vi "Dashboard Main.vi"() -> ()   [LabVIEW 2014]
uses:
  <vilib>/event_ctls.llb/eventvkey.ctl
  <vilib>/Rock Robotics/WPI/Dashboard/WPI_DashboardLogging Global.vi
  <vilib>/Utility/config.llb/Write Key (String).vi
  <vilib>/Utility/config.llb/Write Key (I32).vi
  <vilib>/Utility/config.llb/NI_LVConfig.lvlib
panel:
  in  "TCP":refnum<k5>
  in  "Rec Mode":enum32{"Stop", "Record", "Playback"}(radio)
  in  "Vision":u16(ring) items=["Camera Off", "USB Camera SW", "USB Camera HW", "IP Camera"]
  out "Camera IP":string
  out "Image Message":string="Timeout in Camera Communications"
  in  "Dashboard Tab":T1(tab)
  in  "Camera Settings":T2={"Frame Rate"=30, "Compression"=30, "Size"=1} {"Frame Rate" scale=1.0..30.0; "Size" items=["640x480", "320x240", "160x120"]}
  out "MotorChart R":cluster{"Numeric":dbl, "Numeric":dbl}(graph)
  out "MotorChart L":T3(graph)
  out "MotorSliders R":cluster{"MotorSlide1":dbl, "MotorSlide2":dbl} {"MotorSlide2" scale=-1.0..1.0 scale format="%#_2e"; "MotorSlide1" scale=-1.0..1.0 scale format="%#_2e"}
  out "MotorSliders L":T4 {"MotorSlide4 2" scale=0.0..14.0 scale format="%#_2e"; "MotorSlide2" scale=-1.0..1.0 scale format="%#_2e"; "MotorSlide1" scale=-1.0..1.0 scale format="%#_2e"}
  out "Gyro":dbl(knob) scale=0.0..360.0
  out "JS1 Z":dbl(slide) scale=-1.0..1.0 scale format="%#_2e"
  out "JS1 Graph":cluster{"X":dbl, "Y":dbl}[](graph)
  out "JS1 Buttons":T5
  out "JS2 Z":dbl(slide) scale=-1.0..1.0 scale format="%#_2e"
  out "JS2 Graph":cluster{"X":dbl, "Y":dbl}[](graph)
  out "JS2 Buttons":T5
  out "Mode":T6(ring)=enum."Auto Disabled"
  in  "DB Camera Config":bool
  out "fps":dbl format="%#.1g"
  out "Mbps":dbl format="%#.1g"
  out "Mbps 2":bool
  in  "DB/String 9":string
  in  "DB/String 8":string
  in  "DB/String 7":string
  in  "DB/String 6":string
  in  "DB/String 5":string
  in  "DB/String 4":string
  in  "DB/String 3":string
  in  "DB/String 2":string
  in  "DB/String 1":string
  in  "DB/String 0":string
  in  "DB/Slider 0":dbl(slide) scale=0.0..5.0
  in  "DB/Slider 1":dbl(slide) scale=0.0..5.0
  in  "DB/Slider 2":dbl(slide) scale=0.0..5.0
  in  "DB/Slider 3":dbl(slide) scale=0.0..5.0
  out "DB/LED 3":bool
  out "DB/LED 2":bool
  out "DB/LED 1":bool
  out "DB/LED 0":bool
  in  "DB/Button 3":bool
  in  "DB/Button 2":bool
  in  "DB/Button 1":bool
  in  "DB/Button 0":bool caption="New Name"
  in  "Boolean 2":bool
  in  "Upload code":bool
  out "Speed Value":dbl
  in  "Speed":string
  out "Deadzone Value":dbl
  in  "Deadzone":string
  in  "Upload Code":bool
  in  "Test Slider":dbl(slide) scale=0.0..100.0 scale format="%#_3g"
  in  "On/Off":bool caption="Solenoid"
  in  "Test Name":u16(ring) items=["Select the test to run...", "Example Test", "-------------------------------", "List of tests is built in robot code.", "Replace with your own automated tests."]
  in  "Test Tree":string(tree)
  in  "Motor":cluster{"Value":dbl, "Enable":bool} {"Value" scale=-1.0..1.0 scale format="%#_3g"}
  out "Progress":T7 {"Test Progress" scale=0.0..100.0}
  in  "Rev/Fwd":cluster{"Forward":bool, "Reverse":bool}
  in  "Test Ring":u16(ring) items=["Monochrome", "Color"]
  in  "Listbox":i32(listbox)
  out "Tree":string(tree)
  out "Camera Image":T8(plugin-control)
  out "Boolean":bool
  # "Left"
  # "Front"
  # "Right"
  # "Battery"
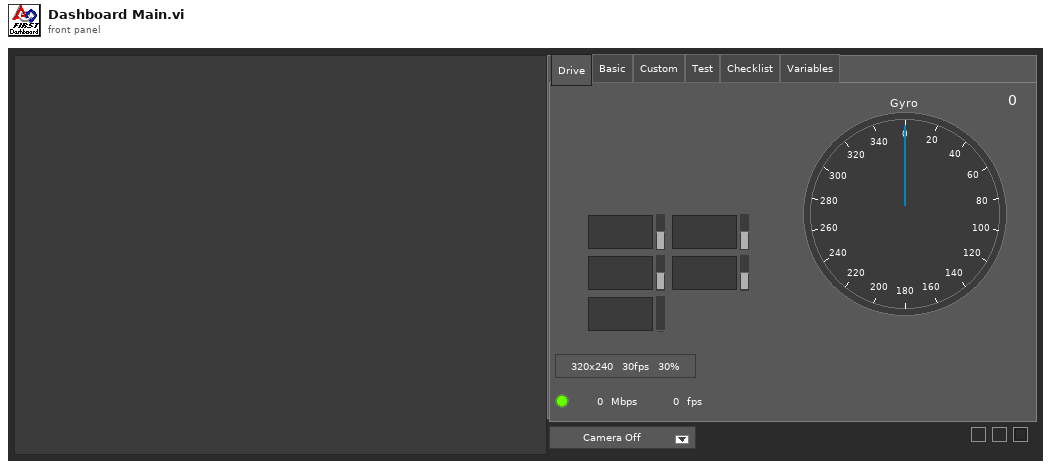
[diagram p1: front panel]
types:
  T1 = enum32{"Drive", "Basic", "Custom", "Test", "Checklist", "Variables"}
  T2 = cluster{"Frame Rate":i32, "Compression":i32, "Size":u16}
  T3 = cluster{"Numeric":dbl, "Numeric":dbl, "Battery V":dbl}
  T4 = cluster{"MotorSlide1":dbl, "MotorSlide2":dbl, "MotorSlide4 2":dbl}
  T5 = cluster{bool, bool, bool, bool, bool, bool, bool, bool, bool, bool, bool, bool}
  T6 = enum8{"Tele-Op Disabled", "Tele-Op Enabled", "Auto Disabled", "Auto Enabled", "Test Disabled", "Test Enabled", "Disconnected", "No Code", "E-Stop"}
  T7 = cluster{"Test Progress":u8, "Test Progress Text":string}
  T8 = typedef "IMAQ Image.ctl" = refnum<image>
  T9 = typedef "Image Type" = u32
  T10 = cluster{"Camera Image":refnum<vi>, "Dashboard Tab":refnum<vi>, "Boolean":refnum<vi>, "Vision":refnum<vi>, "Rec Mode":refnum<vi>, "Test Slider":refnum<vi>, "On/Off ":refnum<vi>, "Test Ring":refnum<vi>, "Rev/Fwd":refnum<vi>, "Test Name":refnum<vi>, "Motor":refnum<vi>, "Progress":refnum<vi>, "CheckList":refnum<vi>, "Tree":refnum<vi>, "Test Tree":refnum<vi>}
  T11 = cluster{"Error Strings":string, "Disable Counts":cluster{u16, u16}, "Rail Faults":cluster{u16, u16, u16}, "Robot IP":string, "DB Mode":u8, "Event Info":cluster{"Name":string, "Type":u8, "Number":u16, "Replay":u8}, "Camera Addr":string}
  T12 = cluster{"Storage":cluster{"Disk Free":u64, "RAM Block":u32, "RAM free":u32}, "CPU Utilization":cluster{"CPU % ISR":sgl, "CPU % Time Crit":sgl, "CPU % Timed Str":sgl, "CPU % High":sgl, "CPU % Above":sgl, "CPU % Normal":sgl, "CPU % Low":sgl}, "CAN":cluster{"% Bus Utilization":sgl, "Bus Off Cnt":u32, "TX_FIFO Full Cnt":u32, "Receive Error Cnt":u8, "Transmit Error Cnt":u8}, "HID":cluster{"HID Outputs":u32, "Rumble Low":u16, "Rumble High":u16}[]}
  T13 = cluster{"Status bits":cluster{"Test Mode":bool, "Autonomous":bool, "Enabled":bool, "Code Start":bool, "Brownout":bool, "Reserved 2":bool, "Reserved 3":bool, "E-Stop":bool}, "Code Trace":cluster{"Disabled":bool, "TeleOp":bool, "Auto":bool, "Test":bool}, "Controller Type":enum16{"unknown", "cRIO", "roboRio"}, "Code?":enum16{"unknown", "noCode", "code"}, "Battery V":dbl}
  T14 = cluster{"Control Bits":cluster{"TestMode":bool, "Autonomous":bool, "Enabled":bool, "FMS Present":bool, bool, bool, bool, "E-Stop":bool}, "Team Station ":u8, "Countdown":sgl, "Joystick Values":cluster{"Axes":dbl[], "Buttons":bool[], "POVs":i16[]}[]}
  T15 = cluster{"Axes":dbl[], "Buttons":bool[], "POVs":i16[]}[]
  T16 = cluster{"Axes":dbl[], "Buttons":bool[], "POVs":i16[]}
  T17 = cluster{"Buttons[0]":bool, "Buttons[1]":bool, "Buttons[2]":bool, "Buttons[3]":bool, "Buttons[4]":bool, "Buttons[5]":bool, "Buttons[6]":bool, "Buttons[7]":bool, "Buttons[8]":bool, "Buttons[9]":bool, "Buttons[10]":bool, "Buttons[11]":bool}
  T18 = typedef "NI_LVConfig.lvlib/Config Data RefNum.ctl" = refnum<k1>
  T19 = cluster{"Operation":enum16{"Update", "Clear"}, "Color Box":u32}[]
  T20 = typedef "eventvkey.ctl" = enum16{"ASCII", "Enter", "Return", "Shift", "Ctrl", "Alt", "Cmd", "Opt", "Caps", "NumLock", "Clear", "Break", "Up", "Down", "Left", "Right", "Insert", "Delete", "Home", "End", "PageUp", "PageDown", "Escape", "Help", "Pause", "ScrollLock", "F1", "F2", "F3", "F4", "F5", "F6", "F7", "F8", "F9", "F10", "F11", "F12", "F13", "F14", "F15", "F16", "F17", "F18", "F19", "F20", "F21", "F22", "F23", "F24", "Play", "VolumeUp", "VolumeDown", "Mute", "Two Byte Char"}
  T21 = cluster{"Image Size":bool, "Image Type":bool, "Pixel Value":bool, "ROI Information":bool, "Zoom Factor":bool}
  T22 = enum8{"Enabled", "Disabled", "Disabled and Grayed Out"}
  T23 = cluster{"Operation":enum16{"Update", "Clear"}, "Color Box":u32}
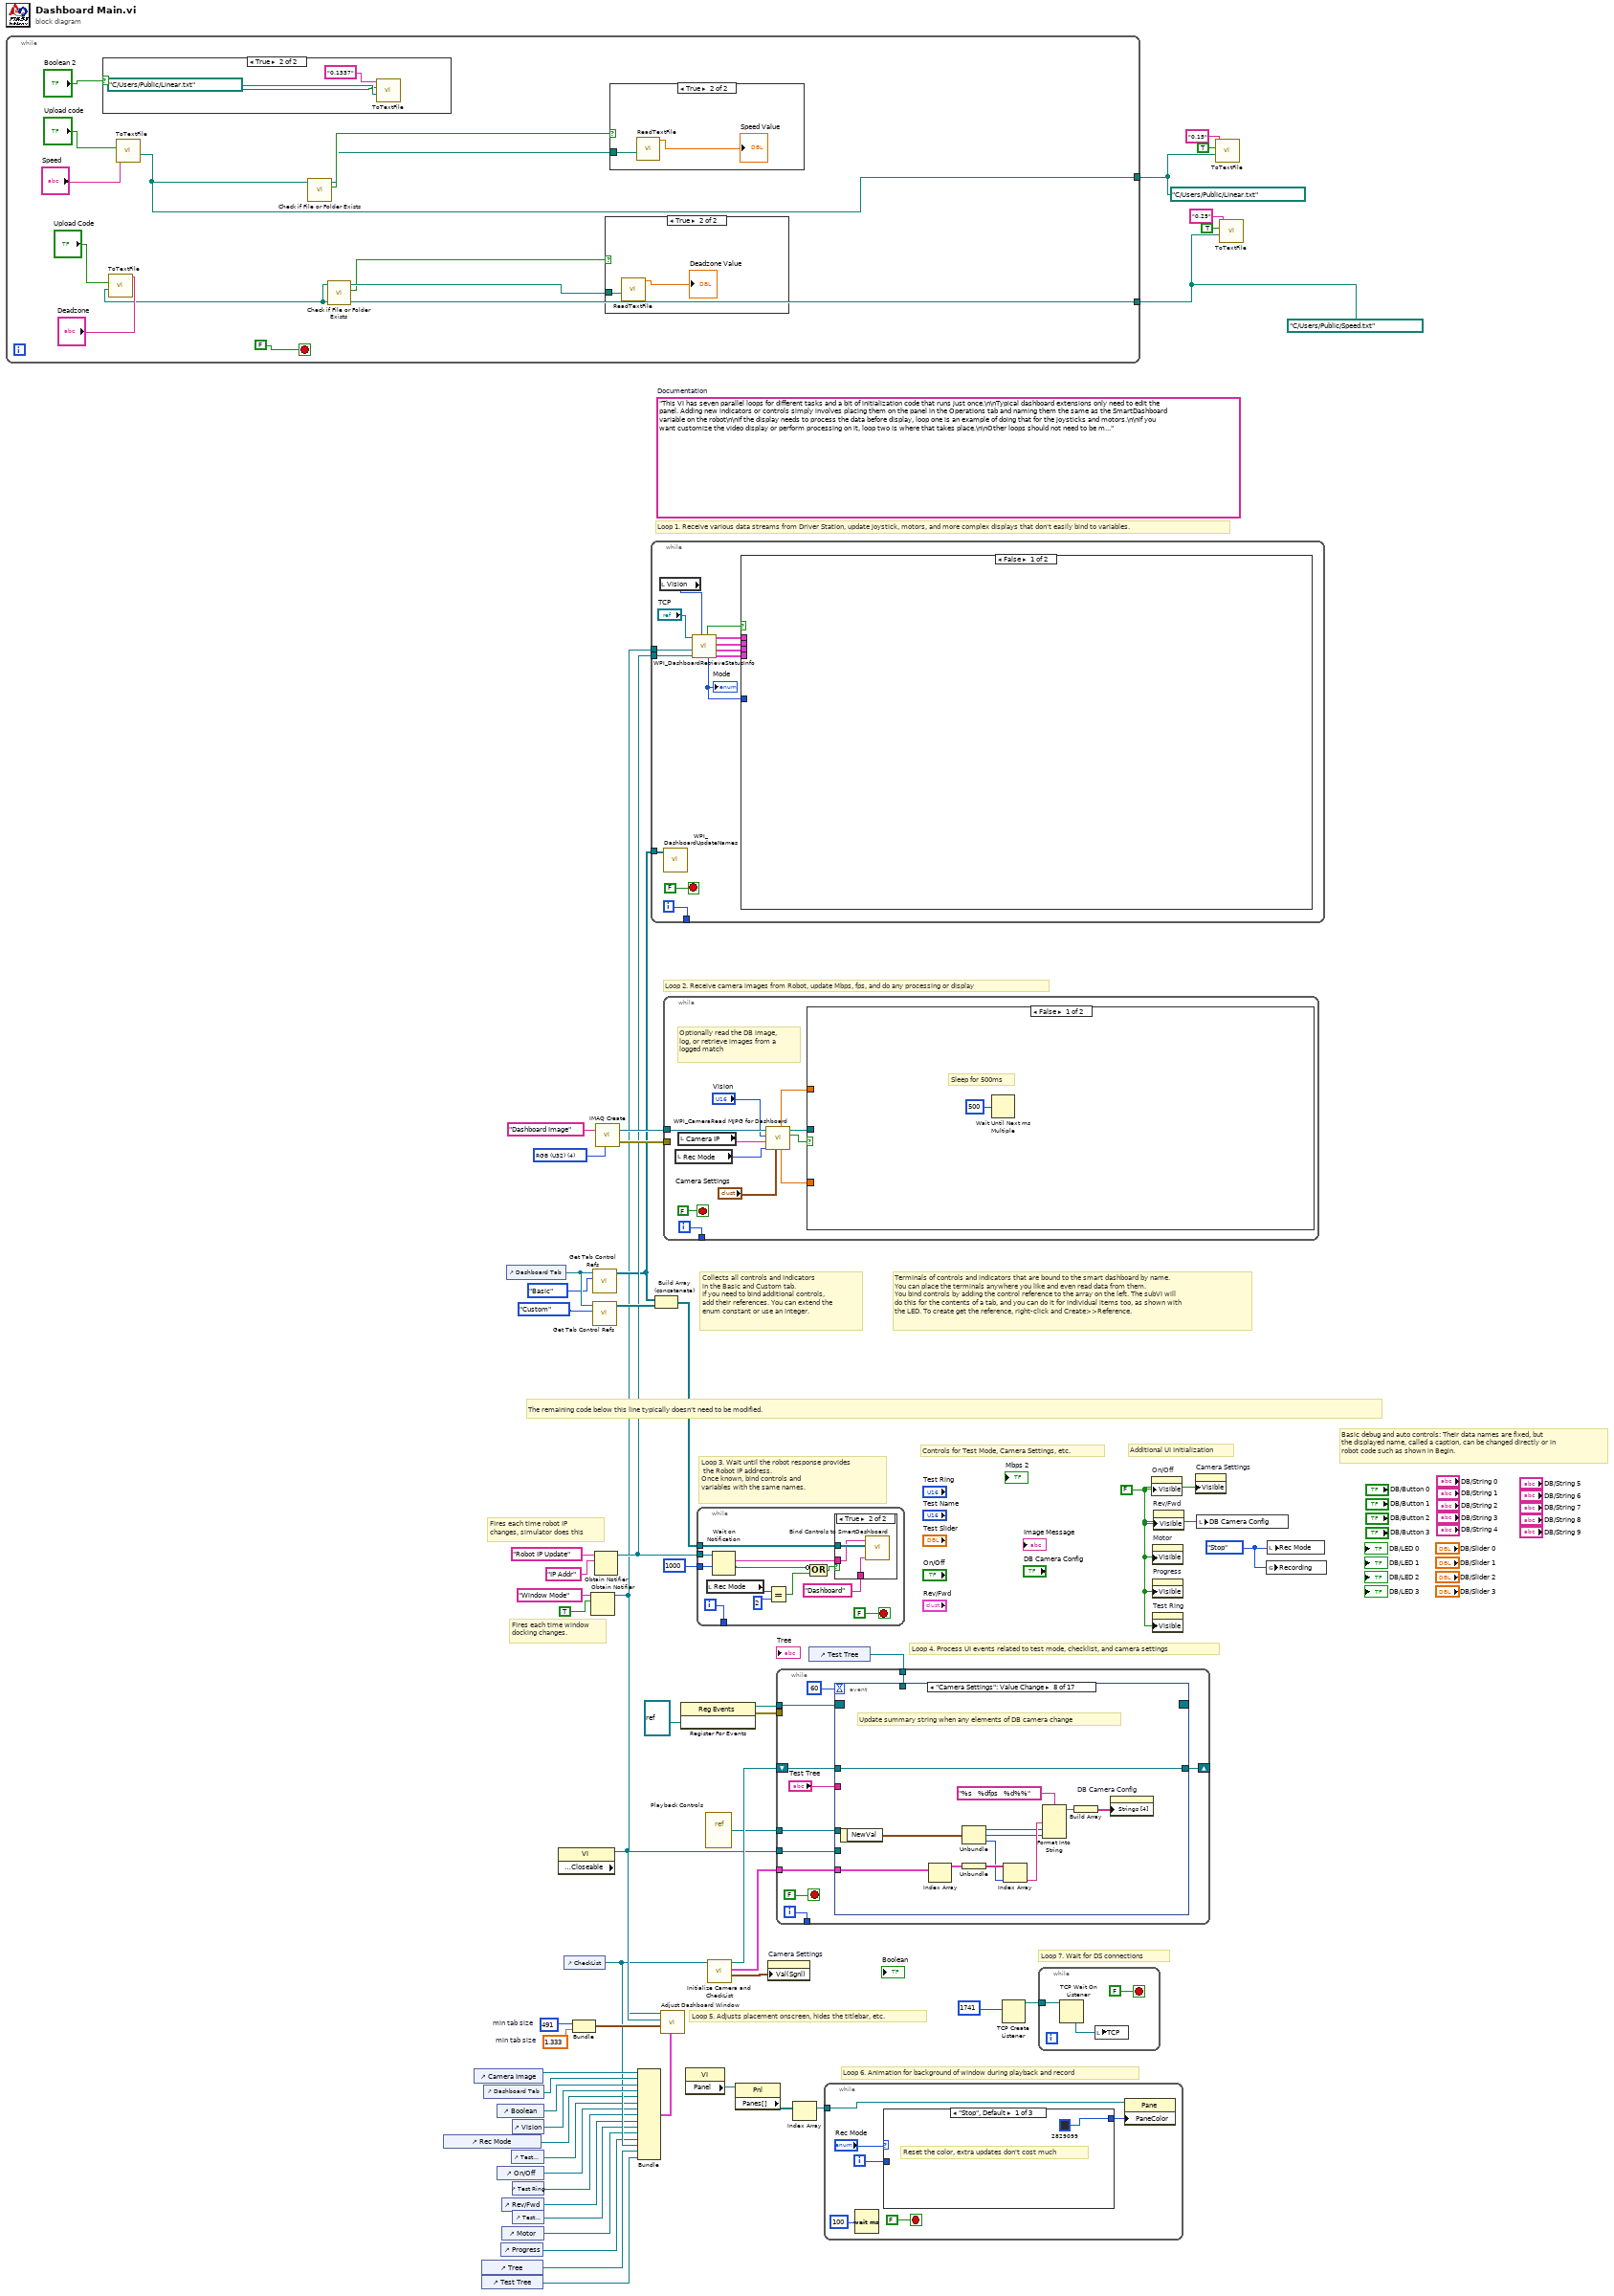
[diagram p0: block diagram]
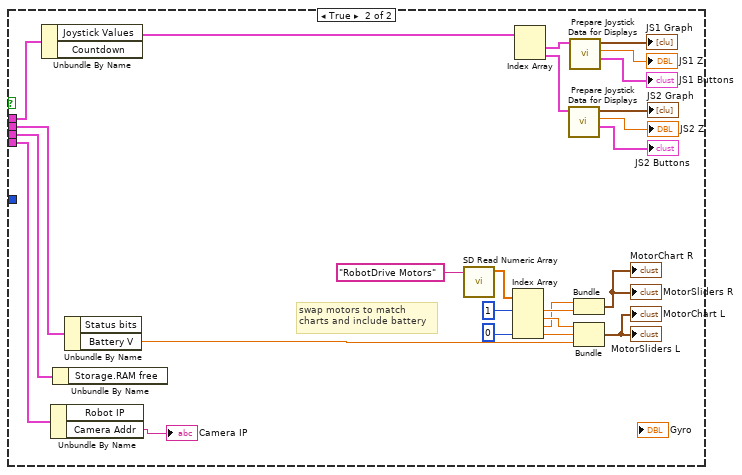
[diagram p5: hidden frame]
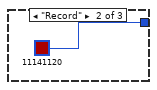
[diagram p6: hidden frame]
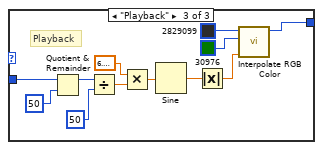
[diagram p7: hidden frame]
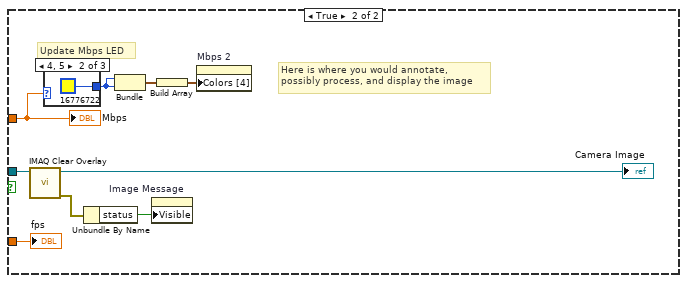
[diagram p9: hidden frame]
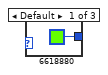
[diagram p10: hidden frame]
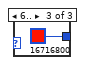
[diagram p11: hidden frame]
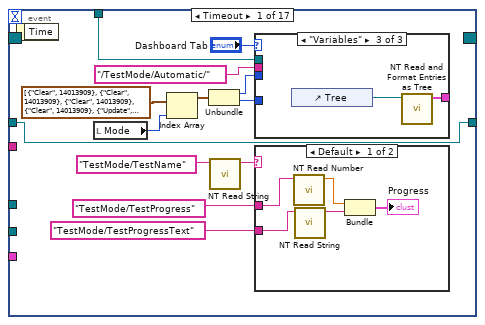
[diagram p12: hidden frame]
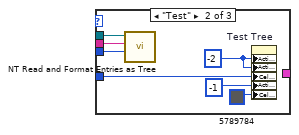
[diagram p14: hidden frame]
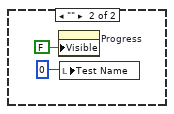
[diagram p15: hidden frame]
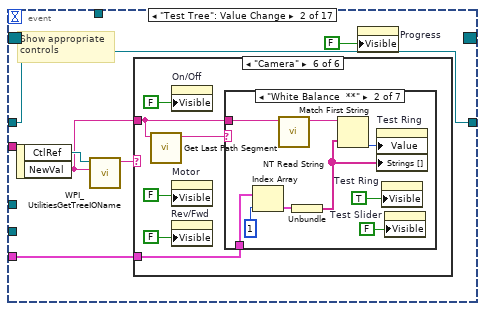
[diagram p16: hidden frame]
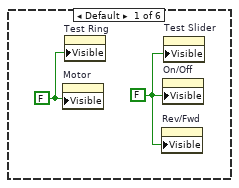
[diagram p17: hidden frame]
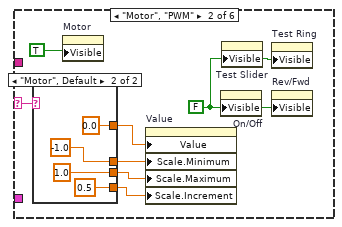
[diagram p18: hidden frame]
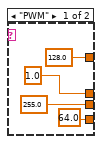
[diagram p19: hidden frame]
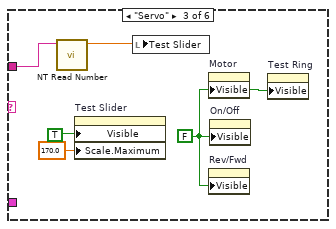
[diagram p20: hidden frame]
diagram:
  w2 = path "C:/Users/Public/Linear.txt" ("file path (use dialog)")
  w1 = path "C:/Users/Public/Speed.txt" ("file path (use dialog)")
  w30 = 491  # min tab size
  w29 = 1.333  # min tab size
  w38 = enum32{"Stop", "Record", "Playback"}."Stop" ("Rec Mode")
  w12 = FALSE ("Visible")
  (unwired) "This VI has seven parallel loops for different tasks and a bit of initialization code that runs just once.\n\nTypical dashboard extensions only need to edit the panel. Adding new indicators or controls simply involves placing them on the panel in the Operations tab and naming them the same as the SmartDashboard variable on the robot\n\nIf the display needs to process the data before display, loop one is an example of doing that for the joysticks and motors.\n\nIf you want customize the video display or perform processing on it, loop two is where that takes place.\n\nOther loops should not need to be modified. They are pretty standard, and document the task they perform."  # Documentation
  w58 = T9 4 items=["Grayscale (U8)", "Grayscale (I16)", "Grayscale (SGL)", "Complex (CSG)", "RGB (U32)", "HSL (U32)", "RGB (U64)"] ("Image Type")
  # "Loop 7. Wait for DS connections"
  # "Basic debug and auto controls: Their data names are fixed, but\nthe displayed name, called a caption, can be changed directly or in\nrobot code such as shown in Begin."
  # "Controls for Test Mode, Camera Settings, etc."
  # "Additional UI Initialization"
  # "Loop 6. Animation for background of window during playback and record"
  # "Fires each time robot IP\nchanges, simulator does this"
  # "Fires each time window\ndocking changes."
  # "Collects all controls and indicators\nin the Basic and Custom tab.\nIf you need to bind additional controls,\nadd their references. You can extend the\nenum constant or use an integer."
  # "The remaining code below this line typically doesn't need to be modified."
  # "Loop 4. Process UI events related to test mode, checklist, and camera settings"
  # "Terminals of controls and indicators that are bound to the smart dashboard by name.\nYou can place the terminals anywhere you like and even read data from them.\nYou bind controls by adding the control reference to the array on the left. The subVI will\ndo this for the contents of a tab, and you can do it for individual items too, as shown with\nthe LED. To create get the reference, right-click and Create>>Reference."
  # "Loop 3. Wait until the robot response provides\n the Robot IP address.\nOnce known, bind controls and\nvariables with the same names."
  # "Loop 5. Adjusts placement onscreen, hides the titlebar, etc."
  # "Loop 1. Receive various data streams from Driver Station, update joystick, motors, and more complex displays that don't easily bind to variables."
  # "Loop 2. Receive camera images from Robot, update Mbps, fps, and do any processing or display"
  n1 = while {
    tunnel: w2 -> [w60]
    tunnel: w1 -> [w59]
    stop <- FALSE stop-if-true
    n2 = case shown="True" "Boolean 2" {
      selector: "Boolean 2" -> [_ w76]
      frame False {
      }
      frame True {
        n3 = call "ToTextFile.vi"("file path (use dialog)"=path "C:/Users/Public/Linear.txt", "Boolean"=w76, "String"="0.1337") -> ()  [unwired: 8 in, 1 out]
      }
    }
    n4 = call "ToTextFile.vi"("file path (use dialog)"=w59, "Boolean"="Upload Code", "String"="Deadzone") -> ()  [unwired: 8 in, 1 out]
    n5 = call "ToTextFile.vi"("file path (use dialog)"=w60, "Boolean"="Upload code", "String"="Speed") -> ()  [unwired: 8 in, 1 out]
    n6 = call <vilib>:"Check if File or Folder Exists.vi"("path"=w60) -> ("file or folder exists?"=w64:bool, "dup path"=w63:path)  [unwired: 8 in, 1 out]
    n7 = call <vilib>:"Check if File or Folder Exists.vi"("path"=w59) -> ("file or folder exists?"=w61:bool, "dup path"=w62:path)  [unwired: 8 in, 1 out]
    n8 = case shown="True" w61 {
      tunnel: w62 -> [_ w71]
      frame False {
      }
      frame True {
        n9 = call "ReadTextFile.vi"("file (use dialog)"=w71) -> ("Double"=→"Deadzone Value":dbl)  [unwired: 9 in, 1 out]
      }
    }
    n10 = case shown="True" w64 {
      tunnel: w63 -> [_ w73]
      frame False {
      }
      frame True {
        n11 = call "ReadTextFile.vi"("file (use dialog)"=w73) -> ("Double"=→"Speed Value":dbl)  [unwired: 9 in, 1 out]
      }
    }
  }
  n12 = control-ref of="Rec Mode"() -> (w18:refnum<vi>)
  n13 = control-ref of="Camera Image"() -> (w33:refnum<vi>)
  n14 = control-ref of="Tree"() -> (w22:refnum<vi>)
  n15 = control-ref of="Test Tree"() -> (w21:refnum<vi>)
  n16 = control-ref of="Dashboard Tab"() -> (w32:refnum<vi>)
  n17 = control-ref of="Boolean"() -> (w27:refnum<vi>)
  n18 = control-ref of="On/Off"() -> (w16:refnum<vi>)
  n19 = control-ref of="Progress"() -> (w13:refnum<vi>)
  n20 = control-ref of="Rev/Fwd"() -> (w14:refnum<vi>)
  n21 = control-ref of="Motor"() -> (w19:refnum<vi>)
  n22 = control-ref of="Dashboard Tab"() -> (w36:refnum<vi>)
  n23 = control-ref of="Test Slider"() -> (w17:refnum<vi>)
  n24 = control-ref of="Vision"() -> (w31:refnum<vi>)
  n25 = control-ref of="Test Ring"() -> (w15:refnum<vi>)
  n26 = control-ref of="Test Name"() -> (w20:refnum<vi>)
  n27 = property class="VI" props=["Front Panel.Closeable"]() -> (reference out=w37:refnum<vi>)  [unwired: 2 in, 2 out]
  n28 = control-ref of="CheckList"() -> (w23:refnum<vi>)
  n29 = Bundle("min tab size"=w30, "min tab size"=w29) -> (w28:cluster{"min tab size":i32, "min tab size":dbl})  [unwired: 1 in]
  n30 = Obtain Notifier(name (unnamed)="Window Mode", notification data type=TRUE) -> (notifier out=w9:refnum<notifier>)  [unwired: 2 in, 2 out]
  n31 = call <vilib>:"Get Tab Control Refs.vi"("Page Index"=T1."Basic" ("Dashboard Tab"), "TabControl in"=w36) -> ("ControlsOnPage"=w10:refnum<vi>[])  [unwired: 9 in]
  n32 = call <vilib>:"Get Tab Control Refs.vi"("Page Index"=T1."Custom" ("Dashboard Tab"), "TabControl in"=w36) -> ("ControlsOnPage"=w35:refnum<vi>[])  [unwired: 9 in]
  n33 = Obtain Notifier(name (unnamed)="Robot IP Update", notification data type="IP Addr" ("name (unnamed)")) -> (notifier out=w11:refnum<notifier>)  [unwired: 2 in, 2 out]
  n34 = call "IMAQ Create"("Image Name"="Dashboard Image", "Image Type"=w58) -> ("New Image"=w56:T8, "error out"=w55:errorcluster)  [unwired: 2 in, 1 out]
  n35 = Bundle("Camera Image"=w33, "Dashboard Tab"=w32, "Boolean"=w27, "Vision"=w31, "Rec Mode"=w18, "Test Slider"=w17, "On/Off"=w16, "Test Ring"=w15, "Rev/Fwd"=w14, "Test Name"=w20, "Motor"=w19, "Progress"=w13, "CheckList"=w23, "Tree"=w22, "Test Tree"=w21) -> (w24:T10)  [unwired: 1 in]
  n36 = while {
    tunnel: [w89] -> _
    tunnel: w11 -> [w83]
    tunnel: w10 -> [w82]
    tunnel: w9 -> [w78]
    i -> [w89]
    stop <- FALSE stop-if-true
    n37 = local read "Vision"() -> (w80:u16)
    n38 = call <vilib>:"WPI_DashboardUpdateNames.vi"("Controls on Tab"=w82) -> ()  [unwired: 11 in]
    n39 = call <vilib>:"WPI_DashboardRetrieveStatusInfo.vi"("Vision"=w80, "Binding Refnum"=w83, "Window Mode Notifier"=w78, "TCP Cnx"="TCP") -> ("Power and Errors"=w84:T11, "Robot Metrics"=w87:T12, "Status Info"=w88:T13, "Control Info"=w85:T14, "Robot Mode"=w81:T6, "Process?"=w86:bool)  [unwired: 2 in]
    "Mode" <- w81
    n40 = case shown="False" w86 {
      tunnel: w88 -> [_ w115]
      tunnel: w87 -> [_ w114]
      tunnel: w85 -> [_ w113]
      tunnel: w84 -> [_ w112]
      tunnel: w81 -> [_ _]
      frame False {
      }
      frame True {
        # "swap motors to match\ncharts and include battery"
        n41 = Unbundle By Name(w113) -> ("Joystick Values"=w100:T15)  [unwired: 1 out]
        n42 = Unbundle By Name(w112) -> ("Camera Addr"=→"Camera IP":string)  [unwired: 1 out]
        n43 = Unbundle By Name(w114) -> ()  [unwired: 1 out]
        n44 = Unbundle By Name(w115) -> ("Battery V"=w101:dbl)  [unwired: 1 out]
        n45 = call <vilib>:"SD Read Numeric Array.vi"("Name"="RobotDrive Motors") -> ("Numeric Array"=w103:dbl[])  [unwired: 8 in, 2 out]
        n46 = Index Array(array=w103, index #1=1, index #4=0) -> (element #1=w107:dbl, element #2=w108:dbl, element #3=w106:dbl, element #4=w111:dbl)  [unwired: 2 in]
        n47 = Index Array(array=w100) -> (element #1=w99:T16, element #2=w94:T16)  [unwired: 2 in]
        n48 = call "Prepare Joystick Data for Displays.vi"("Joystick Values"=w94) -> ("Buttons"=→"JS2 Buttons":T17, "Z Axis"=→"JS2 Z":dbl, "Cartesian Data"=→"JS2 Graph":cluster{"X axis":dbl, "X axis":dbl}[])  [unwired: 8 in]
        n49 = call "Prepare Joystick Data for Displays.vi"("Joystick Values"=w99) -> ("Buttons"=→"JS1 Buttons":T17, "Z Axis"=→"JS1 Z":dbl, "Cartesian Data"=→"JS1 Graph":cluster{"X axis":dbl, "X axis":dbl}[])  [unwired: 8 in]
        n50 = Bundle("Numeric"=w106, "Numeric"=w107) -> (→"MotorChart R" →"MotorSliders R":cluster{"Numeric":dbl, "Numeric":dbl})  [unwired: 1 in]
        n51 = Bundle("Numeric"=w108, "Numeric"=w111, "Battery V"=w101) -> (→"MotorChart L" →"MotorSliders L":T3)  [unwired: 1 in]
      }
    }
  }
  n52 = Build Array (concatenate)(w10, w35) -> (w34:refnum<vi>[])
  n53 = call "Adjust Dashboard Window.vi"("Sizing Refnums"=w24, "Size Constraints"=w28, "VI"=w37, "Notifier in"=w9) -> ()  [unwired: 8 in]
  n54 = while {
    tunnel: w56 -> [w124]
    tunnel: w55 -> [_]
    tunnel: [w125] -> _
    i -> [w125]
    stop <- FALSE stop-if-true
    # "Optionally read the DB image,\nlog, or retrieve images from a\nlogged match"
    n55 = local read "Rec Mode"() -> (w118:enum32{"Stop", "Record", "Playback"})
    n56 = local read "Camera IP"() -> (w116:string)
    n57 = call <vilib>:"WPI_CameraRead MJPG for Dashboard.vi"("Camera Settings"="Camera Settings", "Rec Mode"=w118, "Camera IP"=w116, "Camera Mode"="Vision", "Refnum in"=w124) -> ("Active"=w122:bool, "Refnum out"=w123:T8, "FPS"=w121:dbl, "Bandwidth (Mbps)"=w120:dbl)  [unwired: 3 in]
    n58 = case shown="False" w122 {
      tunnel: w123 -> [_ w131]
      tunnel: w120 -> [_ w130]
      tunnel: w121 -> [_ w128]
      frame False {
        # "Sleep for 500ms"
        n59 = Wait Until Next ms Multiple(millisecond multiple=u32 500) -> ()  [unwired: 1 out]
      }
      frame True {
        # "Here is where you would annotate,\npossibly process, and display the image"
        # "Update Mbps LED"
        n60 = call "IMAQ Clear Overlay"("Image"=w131) -> ("error out"=w135:errorcluster, "Image Out"=→"Camera Image":T8)  [unwired: 2 in, 7 out]
        n61 = case shown="4, 5" w130 {
          tunnel: [u32 6618880 ("Color Box") u32 16776722 ("Color Box") u32 16716800 ("Color Box")] -> w132
          frame Default {
          }
          frame 4, 5 {
          }
          frame 6.. {
          }
        }
        n62 = Unbundle By Name(w135) -> ("status"=w136:bool)
        n63 = Bundle("Color Box"=w132, "Color Box"=w132) -> (w134:cluster{"Color Box":u32, "Color Box":u32})  [unwired: 1 out]
        n64 = property on="Image Message" class="Str"("Visible"=w136) -> ()  [unwired: 2 in, 2 out]
        n65 = Build Array(w134) -> (w133:cluster{"Color Box":u32, "Color Box":u32}[])
        n66 = property on="Mbps 2" class="Bool (strict)"("Colors [4]"=w133) -> ()  [unwired: 2 in, 2 out]
        "Mbps" <- w130
        "fps" <- w128
      }
    }
  }
  n67 = register-events(refnum<vi> refnum) -> (reference out=w42:refnum<event-registration>, error out=w41:errorcluster)  [unwired: 2 in]
  n68 = property class="VI"() -> ("Panel"=w45:refnum<vi>)  [unwired: 2 in, 2 out]
  n69 = while {
    tunnel: w34 -> [w151]
    tunnel: w11 -> [w149]
    tunnel: [w147] -> _
    tunnel: u32 1000 ("milliseconds to wait") -> [w146]
    i -> [w147]
    stop <- FALSE stop-if-true
    n70 = local read "Rec Mode"() -> (w142:enum32{"Stop", "Record", "Playback"})
    n71 = Wait on Notification(notifier=w149, timeout in ms (-1)=w146) -> (notification=w148:string, timed out?=w144:bool)  [unwired: 2 in, 2 out]
    n72 = Equal?(x=w142, y=u16 2 ("Rec Mode")) -> (x = y?=w143:bool)
    n73 = Compound Arithmetic op=OR(invert w144, w143) -> (w145:bool)
    n74 = case shown="True" w145 {
      tunnel: w151 -> [_ w154]
      tunnel: w148 -> [_ w153]
      tunnel: "Dashboard" -> [_ w152]
      frame False {
      }
      frame True {
        n75 = call <vilib>:"Bind Controls to SmartDashboard.vi"("Client Name"=w152, "Bound Control Refs"=w154, "Server IP Address"=w153) -> ()  [unwired: 9 in]
      }
    }
  }
  n76 = vi-ref "Playback Controls.vi"() -> (w43:refnum<vi>)
  n77 = call "Initialize Camera and CheckList.vi"("ListBox in"=w23) -> ("Cluster"=w49:cluster{"value":i32, "value":i32, "index":i32}, "Array"=w50:cluster{string[]}[], "File Refnum"=w48:T18)  [unwired: 8 in]
  n78 = property class="Pnl"(reference=w45) -> ("Panes[]"=w46:refnum<vi>[])  [unwired: 1 in, 2 out]
  n79 = property on="Camera Settings" class="Clust (strict)"("Val(Sgnl)"=w49) -> ()  [unwired: 2 in, 2 out]
  n80 = Index Array(array=w46) -> (element=w44:refnum<vi>)  [unwired: 1 in]
  n81 = control-ref of="Test Tree"() -> (w47:refnum<vi>)
  n82 = while {
    tunnel: w50 -> [w162]
    shift-right: [w161] -> _
    shift-left: w48 -> [w160]
    tunnel: [w159] -> _
    tunnel: w47 -> [w158]
    tunnel: w43 -> [w157]
    tunnel: w42 -> [w156]
    tunnel: w41 -> [_]
    tunnel: w37 -> [w155]
    i -> [w159]
    stop <- FALSE stop-if-true
    n83 = event shown="[7] \"Camera Settings\": Value Change" {
      selector: w156 -> [_ _ _ _ _ _ _ _ _ _ _ _ _ _ _ _ _]
      dyn-events: [_ _ _ _ _ _ _ _ _ _ _ _ _ w400 _ _ _] -> _
      timeout: u32 60 ("milliseconds to wait") -> [_ _ _ _ _ _ _ _ _ _ _ _ _ _ _ _ _]
      tunnel: w158 -> [w174 _ _ _ _ _ _ _ _ _ _ _ _ _ _ _ _]
      tunnel: "Test Tree" -> [_ _ _ _ _ _ _ _ w369 w377 w379 w383 w391 _ _ _ _]
      tunnel: w162 -> [_ w196 _ _ _ _ w333 w363 _ _ _ _ _ _ _ _ _]
      tunnel: [w170 w195 w294 w299 w307 w319 w332 w356 w368 w375 w378 w382 w390 w402 w416 w417 w427] -> w161
      tunnel: w160 -> [w170 w195 w294 w299 w307 w319 w331 w356 w368 w375 w378 w382 w390 w402 w416 w417 w427]
      tunnel: w157 -> [_ _ _ _ _ _ _ _ _ _ _ _ _ w403 _ w420 _]
      tunnel: w155 -> [_ _ _ _ _ _ _ _ _ _ _ _ _ w398 _ _ _]
      event Timeout {
        n84 = event-data() -> ()  [unwired: 1 in, 1 out]
        n85 = local read "Mode"() -> (w173:T6)
        n86 = Index Array(array=T19 [{"Operation"=enum."Clear", "Color Box"=14013909}, {"Operation"=enum."Clear", "Color Box"=14013909}, {"Operation"=enum."Clear", "Color Box"=14013909}, {"Operation"=enum."Clear", "Color Box"=14013909}, {"Operation"=enum."Update", "Color Box"=14013909}, {"Operation"=enum."Update", "Color Box"=16777215}, {"Operation"=enum."Clear", "Color Box"=14013909}, {"Operation"=enum."Clear", "Color Box"=14013909}, {"Operation"=enum."Clear", "Color Box"=14013909}], index=w173) -> (element=w168:T23)
        n87 = Unbundle(w168) -> ("Operation"=w167:enum16{"Update", "Clear"}, "Color Box"=w166:u32)
        n88 = call <vilib>:"NT Read String.vi"("Name"="TestMode/TestName") -> ("String"=w177:string)  [unwired: 9 in, 1 out]
        n89 = case shown="\"Variables\"" "Dashboard Tab" {
          tunnel: w174 -> [_ w185 _]
          tunnel: "/TestMode/Automatic/" ("Name Pattern") -> [_ w184 _]
          tunnel: w167 -> [_ w183 _]
          tunnel: [_ _ w187] -> _
          tunnel: w166 -> [_ w179 _]
          frame "Custom", Default {
          }
          frame "Test" {
            w182 = -2 ("Active Item:Row Number")
            n90 = call <vilib>:"NT Read and Format Entries as Tree.vi"("Operation"=w183, "Name Pattern"=w184, "Tree Refnum"=w185) -> ()  [unwired: 7 in, 2 out]
            n91 = property on="Test Tree" class="Tree (strict)"("Active Item Row Number"=w182, "ActiveColNum"=w182, "CellBG"=w179, "Active Item Row Number"=-1 ("Active Item:Row Number"), "CellBG"=u32 5789784 ("Color Box")) -> ()  [unwired: 2 in, 2 out]
          }
          frame "Variables" {
            n92 = control-ref of="Tree"() -> (w186:refnum<vi>)
            n93 = call <vilib>:"NT Read and Format Entries as Tree.vi"("Tree Refnum"=w186) -> ("Formatted Strings"=w187:cluster{"Name":string, "Value":string}[])  [unwired: 9 in, 1 out]
          }
        }
        n94 = case shown="Default" w177 {
          tunnel: "TestMode/TestProgress" ("Name") -> [w189 _]
          tunnel: "TestMode/TestProgressText" ("Name") -> [w188 _]
          frame Default {
            n95 = call <vilib>:"NT Read Number.vi"("Name"=w189) -> ("Numeric"=w190:dbl)  [unwired: 9 in, 1 out]
            n96 = call <vilib>:"NT Read String.vi"("Name"=w188) -> ("String"=w191:string)  [unwired: 9 in, 1 out]
            n97 = Bundle("Numeric"=w190, "String"=w191) -> (→"Progress":cluster{"Numeric":dbl, "String":string})  [unwired: 1 in]
          }
          frame "" {
            n98 = property on="Progress" class="Clust (strict)"("Visible"=FALSE) -> ()  [unwired: 2 in, 2 out]
            n99 = local write "Test Name"(u16 0) -> ()
          }
        }
      }
      event "Test Tree": Value Change {
        # "Show appropriate\ncontrols"
        n100 = event-data() -> ("CtlRef"=w199:refnum<vi>, "NewVal"=w197:string)  [unwired: 1 in]
        n101 = call <vilib>:"WPI_UtilitiesGetTreeIOName.vi"("NewVal"=w197, "TreeControl in"=w199) -> ("I/O Name"=w200:string)  [unwired: 9 in]
        n102 = case shown="\"Camera\"" w200 {
          selector: w200 -> [_ w207 _ w225 w234 _]
          tunnel: w197 -> [_ _ w222 w224 _ w241]
          tunnel: w196 -> [_ _ _ _ _ w240]
          frame Default {
            w202 = FALSE ("Visible")
            w201 = FALSE ("Visible")
            n103 = property on="Motor" class="Clust (strict)"("Visible"=w201) -> ()  [unwired: 2 in, 2 out]
            n104 = property on="Test Ring" class="Ring (strict)"("Visible"=w201) -> ()  [unwired: 2 in, 2 out]
            n105 = property on="Rev/Fwd" class="Clust (strict)"("Visible"=w202) -> ()  [unwired: 2 in, 2 out]
            n106 = property on="On/Off" class="Bool (strict)"("Visible"=w202) -> ()  [unwired: 2 in, 2 out]
            n107 = property on="Test Slider" class="Slide (strict)"("Visible"=w202) -> ()  [unwired: 2 in, 2 out]
          }
          frame "Motor", "PWM" {
            w208 = FALSE ("Visible")
            n108 = case shown="\"Motor\", Default" w207 {
              tunnel: [1.0 ("Value") -1.0 ("Value")] -> w206
              tunnel: [255.0 ("Value") 1.0 ("Value")] -> w205
              tunnel: [128.0 ("Value") 0.0 ("Value")] -> w204
              tunnel: [64.0 ("Value") 0.5 ("Value")] -> w203
              frame "PWM" {
              }
              frame "Motor", Default {
              }
            }
            n109 = property on="Motor" class="Clust (strict)"("Visible"=TRUE) -> ()  [unwired: 2 in, 2 out]
            n110 = property on="Value" class="Slide (strict)"("Value"=w204, "Scale.Minimum"=w206, "Scale.Maximum"=w205, "Scale.Increment"=w203) -> ()  [unwired: 2 in, 2 out]
            n111 = property on="On/Off" class="Bool (strict)"("Visible"=w208) -> ()  [unwired: 2 in, 2 out]
            n112 = property on="Test Slider" class="Slide (strict)"("Visible"=w208) -> ()  [unwired: 2 in, 2 out]
            n113 = property on="Test Ring" class="Ring (strict)"("Visible"=w208) -> ()  [unwired: 2 in, 2 out]
            n114 = property on="Rev/Fwd" class="Clust (strict)"("Visible"=w208) -> ()  [unwired: 2 in, 2 out]
          }
          frame "Servo" {
            w220 = FALSE ("Visible")
            n115 = call <vilib>:"NT Read Number.vi"("Name"=w222) -> ("Numeric"=w221:dbl)  [unwired: 9 in, 1 out]
            n116 = property on="Test Slider" class="Slide (strict)"("Visible"=TRUE, "Scale.Maximum"=170.0 ("Scale.Range:Maximum")) -> ()  [unwired: 2 in, 2 out]
            n117 = local write "Test Slider"(w221) -> ()
            n118 = property on="Motor" class="Clust (strict)"("Visible"=w220) -> ()  [unwired: 2 in, 2 out]
            n119 = property on="Rev/Fwd" class="Clust (strict)"("Visible"=w220) -> ()  [unwired: 2 in, 2 out]
            n120 = property on="On/Off" class="Bool (strict)"("Visible"=w220) -> ()  [unwired: 2 in, 2 out]
            n121 = property on="Test Ring" class="Ring (strict)"("Visible"=w220) -> ()  [unwired: 2 in, 2 out]
          }
          frame "Relay", "Solenoid" {
            w223 = FALSE ("Visible")
            n122 = property on="Motor" class="Clust (strict)"("Visible"=w223) -> ()  [unwired: 2 in, 2 out]
            n123 = property on="Test Slider" class="Slide (strict)"("Visible"=w223) -> ()  [unwired: 2 in, 2 out]
            n124 = Search and Replace String(input string=w224, search string="/Value  **", replace string="/Direction") -> (result string=w230:string)  [unwired: 5 in, 3 out]
            n125 = property on="Test Ring" class="Ring (strict)"("Visible"=w223) -> ()  [unwired: 2 in, 2 out]
            n126 = call <vilib>:"NT Read String.vi"("Name"=w230) -> ("String"=w228:string)  [unwired: 9 in, 1 out]
            n127 = Equal?(x="Both directions", y=w228) -> (x = y?=w226:bool)
            n128 = Not(x=w226) -> (.not. x?=w227:bool)
            n129 = property on="Rev/Fwd" class="Clust (strict)"("Visible"=w226) -> ()  [unwired: 2 in, 2 out]
            n130 = property on="On/Off" class="Bool (strict)"("Visible"=w227, "Caption.Text"=w225) -> ()  [unwired: 2 in, 2 out]
          }
          frame "Compressor", "Digital Out" {
            w233 = FALSE ("Visible")
            # "Get direction and finish"
            n131 = property on="Motor" class="Clust (strict)"("Visible"=w233) -> ()  [unwired: 2 in, 2 out]
            n132 = property on="Test Slider" class="Slide (strict)"("Visible"=w233) -> ()  [unwired: 2 in, 2 out]
            n133 = property on="Test Ring" class="Ring (strict)"("Visible"=w233) -> ()  [unwired: 2 in, 2 out]
            n134 = property on="On/Off" class="Bool (strict)"("Visible"=TRUE, "Caption.Text"=w234) -> ()  [unwired: 2 in, 2 out]
            n135 = property on="Rev/Fwd" class="Clust (strict)"("Visible"=FALSE) -> ()  [unwired: 2 in, 2 out]
          }
          frame "Camera" {
            n136 = call <vilib>:"Get Last Path Segment.vi"("String in"=w241) -> ("String out"=w242:string)  [unwired: 10 in]
            n137 = property on="On/Off" class="Bool (strict)"("Visible"=FALSE) -> ()  [unwired: 2 in, 2 out]
            n138 = property on="Motor" class="Clust (strict)"("Visible"=FALSE) -> ()  [unwired: 2 in, 2 out]
            n139 = property on="Rev/Fwd" class="Clust (strict)"("Visible"=FALSE) -> ()  [unwired: 2 in, 2 out]
            n140 = case shown="\"White Balance  **\"" w242 {
              tunnel: w241 -> [w248 w257 w266 w275 w284 _ w290]
              tunnel: w240 -> [w246 w254 w263 w272 w281 _ _]
              frame "Size  **" {
                n141 = Index Array(array=w246) -> (element=w245:cluster{string[]})  [unwired: 1 in]
                n142 = call <vilib>:"NT Read String.vi"("Name"=w248) -> ("String"=w247:string)  [unwired: 9 in, 1 out]
                n143 = Unbundle(w245) -> (w243:string[])
                n144 = Match First String(2:w243, 3:w247) -> (0:w244:i32)  [unwired: 1 out]
                n145 = property on="Test Ring" class="Ring (strict)"("Value"=w244, "Strings []"=w243) -> ()  [unwired: 2 in, 2 out]
                n146 = property on="Test Ring" class="Ring (strict)"("Visible"=TRUE) -> ()  [unwired: 2 in, 2 out]
                n147 = property on="Test Slider" class="Slide (strict)"("Visible"=FALSE) -> ()  [unwired: 2 in, 2 out]
              }
              frame "White Balance  **" {
                n148 = Index Array(array=w254, index=1) -> (element=w255:cluster{string[]})
                n149 = call <vilib>:"NT Read String.vi"("Name"=w257) -> ("String"=w256:string)  [unwired: 9 in, 1 out]
                n150 = Unbundle(w255) -> (w252:string[])
                n151 = Match First String(2:w252, 3:w256) -> (0:w251:i32)  [unwired: 1 out]
                n152 = property on="Test Ring" class="Ring (strict)"("Value"=w251, "Strings []"=w252) -> ()  [unwired: 2 in, 2 out]
                n153 = property on="Test Ring" class="Ring (strict)"("Visible"=TRUE) -> ()  [unwired: 2 in, 2 out]
                n154 = property on="Test Slider" class="Slide (strict)"("Visible"=FALSE) -> ()  [unwired: 2 in, 2 out]
              }
              frame "Exposure  **" {
                n155 = Index Array(array=w263, index=2) -> (element=w264:cluster{string[]})
                n156 = call <vilib>:"NT Read String.vi"("Name"=w266) -> ("String"=w265:string)  [unwired: 9 in, 1 out]
                n157 = Unbundle(w264) -> (w260:string[])
                n158 = Match First String(2:w260, 3:w265) -> (0:w261:i32)  [unwired: 1 out]
                n159 = property on="Test Ring" class="Ring (strict)"("Value"=w261, "Strings []"=w260) -> ()  [unwired: 2 in, 2 out]
                n160 = property on="Test Ring" class="Ring (strict)"("Visible"=TRUE) -> ()  [unwired: 2 in, 2 out]
                n161 = property on="Test Slider" class="Slide (strict)"("Visible"=FALSE) -> ()  [unwired: 2 in, 2 out]
              }
              frame "Exposure Priority  **" {
                n162 = Index Array(array=w272, index=3) -> (element=w273:cluster{string[]})
                n163 = call <vilib>:"NT Read String.vi"("Name"=w275) -> ("String"=w274:string)  [unwired: 9 in, 1 out]
                n164 = Unbundle(w273) -> (w269:string[])
                n165 = Match First String(2:w269, 3:w274) -> (0:w270:i32)  [unwired: 1 out]
                n166 = property on="Test Ring" class="Ring (strict)"("Value"=w270, "Strings []"=w269) -> ()  [unwired: 2 in, 2 out]
                n167 = property on="Test Ring" class="Ring (strict)"("Visible"=TRUE) -> ()  [unwired: 2 in, 2 out]
                n168 = property on="Test Slider" class="Slide (strict)"("Visible"=FALSE) -> ()  [unwired: 2 in, 2 out]
              }
              frame "Color Enable  **" {
                n169 = Index Array(array=w281, index=4) -> (element=w282:cluster{string[]})
                n170 = call <vilib>:"NT Read String.vi"("Name"=w284) -> ("String"=w283:string)  [unwired: 9 in, 1 out]
                n171 = Unbundle(w282) -> (w278:string[])
                n172 = Match First String(2:w278, 3:w283) -> (0:w279:i32)  [unwired: 1 out]
                n173 = property on="Test Ring" class="Ring (strict)"("Value"=w279, "Strings []"=w278) -> ()  [unwired: 2 in, 2 out]
                n174 = property on="Test Ring" class="Ring (strict)"("Visible"=TRUE) -> ()  [unwired: 2 in, 2 out]
                n175 = property on="Test Slider" class="Slide (strict)"("Visible"=FALSE) -> ()  [unwired: 2 in, 2 out]
              }
              frame Default {
                n176 = property on="Test Ring" class="Ring (strict)"("Visible"=FALSE) -> ()  [unwired: 2 in, 2 out]
                n177 = property on="Test Slider" class="Slide (strict)"("Visible"=FALSE) -> ()  [unwired: 2 in, 2 out]
              }
              frame "Brightness  **", "Color Level  **", "Compression  **", "FPS  **", "Sharpness  **" {
                n178 = call <vilib>:"NT Read Number.vi"("Name"=w290) -> ("Numeric"=w289:dbl)  [unwired: 9 in, 1 out]
                n179 = local write "Test Slider"(w289) -> ()
                n180 = property on="Test Slider" class="Slide (strict)"("Visible"=TRUE, "Scale.Maximum"=100.0 ("Scale.Range:Maximum")) -> ()  [unwired: 2 in, 2 out]
                n181 = property on="Test Ring" class="Ring (strict)"("Visible"=FALSE) -> ()  [unwired: 2 in, 2 out]
              }
            }
          }
        }
        n182 = property on="Progress" class="Clust (strict)"("Visible"=FALSE) -> ()  [unwired: 2 in, 2 out]
      }
      event "Test Name": Mouse Enter {
        # "Populate the ring with the list of tests"
        n183 = event-data() -> ()  [unwired: 1 in, 1 out]
        n184 = call <vilib>:"NT Read String Array.vi"("Name"="TestMode/TestList") -> ("String Array"=w298:string[])  [unwired: 9 in, 1 out]
        n185 = Build Array (concatenate)("Select the test to run...", w298) -> (w297:string[])
        n186 = property on="Test Name" class="Ring (strict)"("Strings []"=w297) -> ()  [unwired: 2 in, 2 out]
      }
      event "Test Name": Value Change {
        w300 = FALSE ("Visible")
        # "Tell the robot the test name to run"
        n187 = event-data() -> ("NewVal"=w304:u16)  [unwired: 1 in]
        n188 = property on="Test Name" class="Ring (strict)"() -> ("Strings []"=w305:string[])  [unwired: 2 in, 2 out]
        n189 = local write "Progress"(T7 {"Test Progress"=0, "Test Progress Text"=""} ("Progress")) -> ()
        n190 = Index Array(array=w305, index=w304) -> (element=w303:string)
        n191 = call <vilib>:"NT Write String.vi"("String"=w303, "Name"="TestMode/TestName") -> ()  [unwired: 9 in, 1 out]
        n192 = property on="Progress" class="Clust (strict)"("Visible"=TRUE) -> ()  [unwired: 2 in, 2 out]
        n193 = property on="Motor" class="Clust (strict)"("Visible"=w300) -> ()  [unwired: 2 in, 2 out]
        n194 = property on="Test Slider" class="Slide (strict)"("Visible"=w300) -> ()  [unwired: 2 in, 2 out]
        n195 = property on="On/Off" class="Bool (strict)"("Visible"=w300) -> ()  [unwired: 2 in, 2 out]
        n196 = property on="Rev/Fwd" class="Clust (strict)"("Visible"=w300) -> ()  [unwired: 2 in, 2 out]
        n197 = property on="Test Ring" class="Ring (strict)"("Visible"=w300) -> ()  [unwired: 2 in, 2 out]
      }
      event "Listbox": Double Click {
        # "Shift clears all"
        # "Update symbols on the listbox"
        n198 = event-data() -> ("PlatMods.Shift"=w308:bool, "Row"=w310:i32)  [unwired: 1 in]
        n199 = case shown="True" w308 {
          tunnel: w310 -> [w314 _]
          tunnel: 1 -> [w313 _]
          frame False {
            n200 = property on="Listbox" class="LstBox (strict)"() -> ("Item Symbols"=w312:i32[])  [unwired: 2 in, 2 out]
            n201 = Replace Array Subset(array=w312, new element=w313, index=w314) -> (w311:i32[])
            n202 = property on="Listbox" class="LstBox (strict)"("Item Symbols"=w311) -> ()  [unwired: 2 in, 2 out]
          }
          frame True {
            w315 = 0 ("Top Row")
            n203 = property on="Listbox" class="LstBox (strict)"() -> ("Number of Rows"=w317:u32)  [unwired: 2 in, 2 out]
            n204 = Initialize Array(0, w317) -> (w316:i32[])
            n205 = property on="Listbox" class="LstBox (strict)"("Top Row"=w315, "Value"=w315, "Item Symbols"=w316) -> ()  [unwired: 2 in, 2 out]
          }
        }
      }
      event "Listbox": Key Down {
        # "Update symbols on the listbox\nLeft and right keys check and uncheck"
        n206 = event-data() -> ("VKey"=w321:T20)  [unwired: 1 in]
        n207 = case shown="\"Left\", \"Right\"" w321 {
          selector: w321 -> [w326 _]
          tunnel: eventvkey."Left" ("VKey") -> [w324 _]
          frame "Left", "Right" {
            n208 = Equal?(x=w324, y=w326) -> (x = y?=w325:bool)
            n209 = Select(t=0, s=w325, f=1) -> (s? t:f=w327:i32)
            n210 = property on="Listbox" class="LstBox (strict)"() -> ("Item Symbols"=w330:i32[])  [unwired: 2 in, 2 out]
            n211 = Replace Array Subset(array=w330, new element=w327, index="Listbox") -> (w329:i32[])
            n212 = property on="Listbox" class="LstBox (strict)"("Item Symbols"=w329) -> ()  [unwired: 2 in, 2 out]
          }
          frame Default {
          }
        }
      }
      event "DB Camera Config": Value Change {
        # "Show or hide the cluster of controls, store in ini file"
        n213 = event-data() -> ("NewVal"=w334:bool)  [unwired: 1 in]
        n214 = case shown="False" w334 {
          tunnel: w333 -> [w343 _]
          tunnel: [w336 w354] -> w332
          tunnel: w331 -> [w335 w354]
          frame False {
            w350 = "Camera"
            w353 = FALSE ("Visible")
            n215 = local read "Camera Settings"() -> (w342:T2)
            n216 = Index Array(array=w343) -> (element=w346:cluster{string[]})  [unwired: 1 in]
            n217 = Unbundle(w342) -> ("Frame Rate"=w341:i32, "Compression"=w340:i32, "Size"=w344:u16)
            n218 = Unbundle(w346) -> (w345:string[])
            n219 = Index Array(array=w345, index=w344) -> (element=w339:string)
            n220 = call-poly <vilib>:"Write Key.vi"("section"=w350, "value"=w339, "key"="Size", "refnum"=w335) -> ("refnum out"=w352:T18)  [unwired: 2 in, 5 out]
            n221 = call-poly <vilib>:"Write Key.vi"("section"=w350, "value"=w341, "key"="FrameRate", "refnum"=w352) -> ("refnum out"=w351:T18)  [unwired: 1 in, 6 out]
            n222 = property on="Camera Settings" class="Clust (strict)"("Visible"=w353) -> ()  [unwired: 2 in, 2 out]
            n223 = local write "DB Camera Config"(w353) -> ()
            n224 = call-poly <vilib>:"Write Key.vi"("section"=w350, "value"=w340, "key"="Compression", "refnum"=w351) -> ("refnum out"=w337:T18)  [unwired: 1 in, 6 out]
            n225 = call <vilib>:"Close Config Data.vi"("refnum"=w337) -> ("file path"=w338:path)  [unwired: 2 in, 8 out]
            n226 = call <vilib>:"Open Config Data.vi"("configuration file path"=w338) -> ("refnum"=w336:T18)  [unwired: 8 in, 2 out]
          }
          frame True {
            n227 = property on="Camera Settings" class="Clust (strict)"("Visible"=TRUE) -> ()  [unwired: 2 in, 2 out]
          }
        }
      }
      event "Camera Settings": Value Change {
        # "Update summary string when any elements of DB camera change"
        n228 = event-data() -> ("NewVal"=w367:T2)  [unwired: 1 in]
        n229 = Index Array(array=w363) -> (element=w362:cluster{string[]})  [unwired: 1 in]
        n230 = Unbundle(w367) -> ("Frame Rate"=w358:i32, "Compression"=w357:i32, "Size"=w360:u16)
        n231 = Unbundle(w362) -> (w361:string[])
        n232 = Index Array(array=w361, index=w360) -> (element=w359:string)
        n233 = Format Into String(format string="%s   %dfps   %d%%", w359, w358, w357) -> (resulting string=w364:string)  [unwired: 2 in, 1 out]
        n234 = Build Array(w364) -> (w365:string[])
        n235 = property on="DB Camera Config" class="Bool (strict)"("Strings [4]"=w365) -> ()  [unwired: 2 in, 2 out]
      }
      event "Motor.Enable": Value Change {
        # "When the test mode otor enable helper is set, update that\ntree row item's value"
        n236 = event-data() -> ("NewVal"=w373:bool)  [unwired: 1 in]
        n237 = Unbundle("Motor") -> ("Value"=w372:dbl)  [unwired: 1 out]
        n238 = Select(t=w372, s=w373, f=0.0) -> (s? t:f=w370:dbl)
        n239 = call <vilib>:"NT Write Number.vi"("Numeric"=w370, "Name"=w369) -> ()  [unwired: 9 in, 1 out]
      }
      event "Test Slider": Value Change {
        # "When the test mode slider helper is set, update that\ntree row item's value"
        n240 = event-data() -> ("NewVal"=w376:dbl)  [unwired: 1 in]
        n241 = call <vilib>:"NT Write Number.vi"("Numeric"=w376, "Name"=w377) -> ()  [unwired: 9 in, 1 out]
      }
      event "On/Off": Value Change {
        # "When the test mode on/off helper value is set, update that\ntree row item's value"
        n242 = event-data() -> ("NewVal"=w381:bool)  [unwired: 1 in]
        n243 = Boolean To (0,1)(Boolean=w381) -> (0, 1=w380:i16)
        n244 = call <vilib>:"NT Write Number.vi"("Numeric"=w380, "Name"=w379) -> ()  [unwired: 9 in, 1 out]
      }
      event "Rev/Fwd": Value Change {
        # "When the test mode helper value for relays is set, update that\ntree row item's value"
        n245 = event-data() -> ("NewVal.Forward"=w389:bool, "NewVal.Reverse"=w388:bool)  [unwired: 1 in]
        n246 = Boolean To (0,1)(Boolean=w389) -> (0, 1=w385:i16)
        n247 = Boolean To (0,1)(Boolean=w388) -> (0, 1=w387:i16)
        n248 = Negate(x=w387) -> (-x=w386:i16)
        n249 = Add(x=w385, y=w386) -> (x+y=w384:i16)
        n250 = call <vilib>:"NT Write Number.vi"("Numeric"=w384, "Name"=w383) -> ()  [unwired: 9 in, 1 out]
      }
      event "Test Ring": Value Change {
        # "When a test mode helper value is selected from the ring,\nset the tree item's variable to the string value"
        n251 = event-data() -> ("NewVal"=w393:u16)  [unwired: 1 in]
        n252 = property on="Test Ring" class="Ring (strict)"() -> ("Strings []"=w394:string[])  [unwired: 2 in, 2 out]
        n253 = Index Array(array=w394, index=w393) -> (element=w392:string)
        n254 = call <vilib>:"NT Write String.vi"("String"=w392, "Name"=w391) -> ()  [unwired: 9 in, 1 out]
      }
      event "Rec Mode": Value Change {
        # "Update globals for recording mode and path to read log from.\nClear when logging and let NetworkTables set path for vision to\nuse."
        n255 = event-data() -> ("NewVal"=w404:enum32{"Stop", "Record", "Playback"})  [unwired: 1 in]
        n256 = global write "WPI_DashboardLogging Global.vi" "Logging Filename"(path "") -> ()
        n257 = case shown="\"Playback\"" w404 {
          tunnel: w403 -> [_ w406 w414]
          tunnel: [_ _ w413] -> w400
          tunnel: [_ _ w412] -> _
          tunnel: w398 -> [_ _ w410]
          tunnel: cluster{i32, i32} {-250, 170} -> [_ _ w409]
          tunnel: [_ _ T21 {"Image Size"=TRUE, "Image Type"=TRUE, "Pixel Value"=TRUE, "ROI Information"=TRUE, "Zoom Factor"=FALSE} ("Image Information Shown:All Elements")] -> w396
          tunnel: [_ _ TRUE ("Zoom Factor")] -> w395
          frame Default {
          }
          frame "Stop", "Record" {
            # "Place Window too"
            n258 = invoke class="VI" method="FP.Close"(reference=w406) -> (reference out=w405:refnum<vi>)  [unwired: 2 in, 2 out]
            n259 = invoke class="VI" method="Abort VI"(reference=w405) -> ()  [unwired: 2 in, 3 out]
          }
          frame "Playback" {
            n260 = call "Open Playback Panel.vi"("Offset"=w409, "DB VI Ref"=w410, "Playback in"=w414) -> ("Playback out"=w411:refnum<vi>)  [unwired: 8 in]
            n261 = register-events(w411) -> (reference out=w413:refnum<event-registration>, error out=w412:errorcluster)  [unwired: 2 in]
          }
        }
        n262 = global write "WPI_DashboardLogging Global.vi" "Recording"(w404) -> ()
        n263 = property on="Camera Image" class="ImageControl"("Image Information Shown"=w396, "Image Information Visible"=w395) -> ()  [unwired: 2 in, 2 out]
        n264 = call <vilib>:"WPI_DashboardNT Log FieldName Cache.vi"("Operation"=enum16{"Lookup/Add", "Index", "Clear"}."Clear") -> ()  [unwired: 8 in, 3 out]
      }
      event Panel Close {
        w415 = enum32{"Stop", "Record", "Playback"}."Stop" ("Rec Mode")
        # "Playback window has been closed, abort"
        n265 = event-data() -> ()  [unwired: 1 in, 4 out]
        n266 = local write "Rec Mode"(w415) -> ()
        n267 = global write "WPI_DashboardLogging Global.vi" "Recording"(w415) -> ()
      }
      event Panel Close {
        # "Abort playback window and ourself"
        n268 = event-data() -> ()  [unwired: 1 in, 4 out]
        n269 = invoke class="VI" method="FP.Close"(reference=w420) -> (reference out=w419:refnum<vi>)  [unwired: 2 in, 2 out]
        n270 = invoke class="VI" method="Abort VI"(reference=w419) -> (error out=w418:errorcluster)  [unwired: 2 in, 2 out]
        n271 = invoke class="VI" method="Abort VI"(error in=w418) -> ()  [unwired: 2 in, 3 out]
      }
      event "Vision": Value Change {
        # "Enable/Disable Compression slider.\nHW USB is hard-coded into the camera"
        n272 = event-data() -> ("NewVal"=w426:u16)  [unwired: 1 in]
        n273 = Equal?(x=w426, y=u32 2 ("milliseconds to wait")) -> (x = y?=w424:bool)
        n274 = Select(t=T22."Disabled and Grayed Out" ("Disabled"), s=w424, f=T22."Enabled" ("Disabled")) -> (s? t:f=w421:T22)
        n275 = property on="Compression" class="Slide (strict)"("DisabledEnum"=w421) -> ()  [unwired: 2 in, 2 out]
      }
    }
  }
  n276 = while {
    tunnel: w44 -> [w429]
    i -> [w432]
    stop <- FALSE stop-if-true
    n277 = Wait (ms)(milliseconds to wait=u32 100) -> ()  [unwired: 1 out]
    n278 = case shown="\"Stop\", Default" "Rec Mode" {
      tunnel: w432 -> [_ _ w447]
      tunnel: [u32 2829099 ("Base Color") u32 11141120 ("Target Color") w436] -> w428
      frame "Stop", Default {
        # "Reset the color, extra updates don't cost much"
      }
      frame "Record" {
      }
      frame "Playback" {
        # "Playback"
        n279 = Quotient & Remainder(x=w447, y=u32 50 ("milliseconds to wait")) -> (x-y*floor(x/y)=w443:u32)  [unwired: 1 out]
        n280 = Divide(x=w443, y=u32 50 ("milliseconds to wait")) -> (x/y=w440:dbl)
        n281 = Multiply(x=6.283185307179586, y=w440) -> (x*y=w445:dbl)
        n282 = Sine(x=w445) -> (sin(x)=w444:dbl)
        n283 = Absolute Value(x=w444) -> (abs(x)=w437:dbl)
        n284 = call "Interpolate RGB Color.vi"("Proportion"=w437, "Target Color"=u32 30976, "Base Color"=u32 2829099) -> ("Result Color"=w436:u32)  [unwired: 8 in]
      }
    }
    n285 = property class="Pane"(reference=w429, "PaneColor"=w428) -> ()  [unwired: 1 in, 2 out]
  }
  n286 = TCP Create Listener(10:u16 1741 ("timeout ms (25000)")) -> (3:w7:refnum<k5>)  [unwired: 4 in, 2 out]
  n287 = while {
    tunnel: w7 -> [w449]
    stop <- FALSE stop-if-true
    n288 = TCP Wait On Listener(11:w449) -> (4:w448:refnum<k5>)  [unwired: 3 in, 4 out]
    n289 = local write "TCP"(w448) -> ()
  }
  n290 = property on="On/Off" class="Bool (strict)"("Visible"=w12) -> ()  [unwired: 2 in, 2 out]
  n291 = property on="Motor" class="Clust (strict)"("Visible"=w12) -> ()  [unwired: 2 in, 2 out]
  n292 = property on="Progress" class="Clust (strict)"("Visible"=w12) -> ()  [unwired: 2 in, 2 out]
  n293 = property on="Test Ring" class="Ring (strict)"("Visible"=w12) -> ()  [unwired: 2 in, 2 out]
  n294 = property on="Rev/Fwd" class="Clust (strict)"("Visible"=w12) -> ()  [unwired: 2 in, 2 out]
  n295 = property on="Camera Settings" class="Clust (strict)"("Visible"=w12) -> ()  [unwired: 2 in, 2 out]
  n296 = local write "DB Camera Config"(w12) -> ()
  n297 = call "ToTextFile.vi"("file path (use dialog)"=w2, "Boolean"=TRUE, "String"="0.15") -> ()  [unwired: 8 in, 1 out]
  n298 = call "ToTextFile.vi"("file path (use dialog)"=w1, "Boolean"=TRUE, "String"="0.25") -> ()  [unwired: 8 in, 1 out]
  n299 = global write "WPI_DashboardLogging Global.vi" "Recording"(w38) -> ()
  n300 = local write "Rec Mode"(w38) -> ()
